vi "write_signal_hdf5.vi"(7 "Index":i32, 8 "error in":errorcluster, 10 "Save Path":path, 11 "Signal array":T2[](array[typedef])) -> (0 "error out":errorcluster, 3 "Signal Processing:":T4={"Integer Timestamp"=0, "Dust Event ID"=0, "Role ID"=enum."First_Detector", "Data"=[], "Signal Length"=0, "dt"=0.0, "Offset"=0.0, "Hardware ID"=enum."CSA 1"})   [LabVIEW 2013]
uses:
  <userlib>/Accelerator/User Interface/Controls/Post_Signal.ctl
  <userlib>/Accelerator/User Interface/Controls/Role ID.ctl
  <userlib>/Accelerator/User Interface/Controls/Hardware ID.ctl
  <userlib>/Accelerator/User Interface/Controls/Signal.ctl
  <vilib>/addons/h5labview/polymorph/H5D_write_var.vi
  <vilib>/addons/h5labview/H5Dataset.lvlib
  <vilib>/addons/h5labview/H5Attrib.lvlib
  <vilib>/addons/h5labview/H5File.lvlib
panel:
  out "concatenated string":string
  out "Role ID":T1
  # "Signal"
  # "Signal"
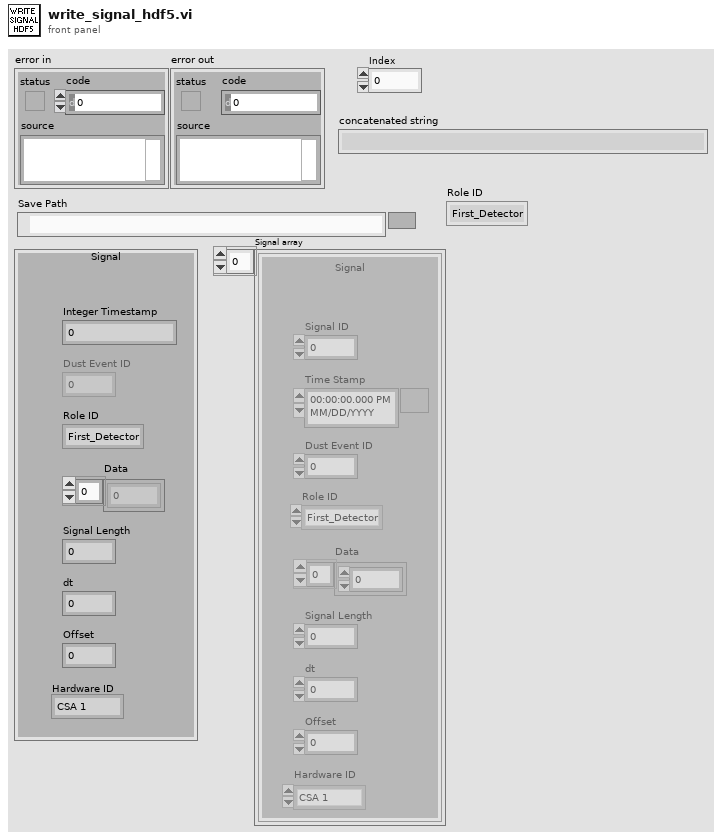
[diagram p1: front panel]
types:
  T1 = typedef "Role ID.ctl" = enum16{"First_Detector", "Second_Detector", "Third_Detector", "LeCroy_CH1", "LeCroy_CH2", "LeCroy_CH3", "LeCroy_CH4", "PSU", "DCS 1", "DCS 2"}
  T2 = typedef "Signal.ctl" = cluster{"Signal ID":i64, "Time Stamp":timestamp, "Dust Event ID":i64, "Role ID":T1, "Data":sgl[], "Signal Length":i32, "dt":sgl, "Offset":dbl, "Hardware ID":T3}
  T3 = typedef "Hardware ID.ctl" = enum16{"Unknown", "CSA 1", "CSA 2", "CSA 3", "CSA 4", "CSA 5", "CSA 6", "DCS 1", "DCS 2"}
  T4 = typedef "Post_Signal.ctl" = cluster{"Integer Timestamp":i64, "Dust Event ID":i64, "Role ID":T1, "Data":sgl[], "Signal Length":i32, "dt":sgl, "Offset":dbl, "Hardware ID":T3}
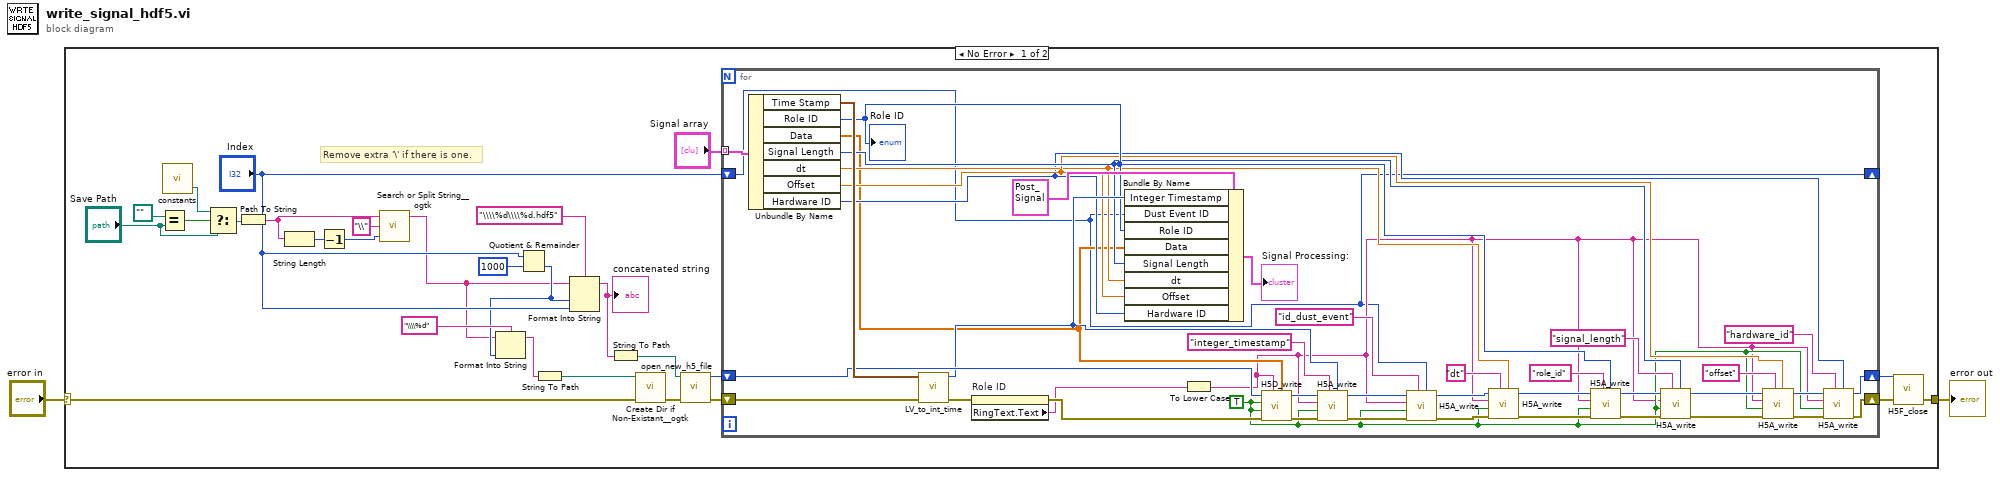
[diagram p0: block diagram]
diagram:
  n1 = case shown="No Error" "error in" {
    selector: "error in" -> [w3 w72]
    tunnel: [w5 w72] -> w1
    frame No Error {
      # "Remove extra '\\' if there is one."
      n2 = Equal?(x=path "" ("Save Path"), y="Save Path") -> (x = y?=w24:bool)
      n3 = call <userlib>:"constants.vi"() -> ("file path for Processed Signal .hdf5 files"=w4:path)  [unwired: 3 in, 2 out]
      n4 = Select(t=w4, s=w24, f="Save Path") -> (s? t:f=w26:path)
      n5 = Path To String(path=w26) -> (string=w9:string)
      n6 = String Length(string=w9) -> (length=w10:i32)
      n7 = Decrement(x=w10) -> (x-1=w11:i32)
      n8 = call <userlib>:"Search or Split String__ogtk.vi"("offset (0)"=w11, "search string/char (-)"="\\", "string"=w9) -> ("substring before match"=w8:string)  [unwired: 2 out]
      n9 = Quotient & Remainder(x="Index", y=1000) -> (floor(x/y)=w15:i32)  [unwired: 1 out]
      n10 = Format Into String(format string="\\\\%d", initial string=w8, w15) -> (resulting string=w16:string)  [unwired: 1 in, 1 out]
      n11 = String To Path(string=w16) -> (path=w13:path)
      n12 = Format Into String(format string="\\\\%d\\\\%d.hdf5", initial string=w8, w15, "Index") -> (resulting string=w19:string)  [unwired: 1 in, 1 out]
      "concatenated string" <- w19
      n13 = String To Path(string=w19) -> (path=w22:path)
      n14 = call <userlib>:"Create Dir if Non-Existant__ogtk.vi"("error in (no error)"=w3, "Directory Path"=w13) -> ("error out"=w14:errorcluster)  [unwired: 7 in, 2 out]
      n15 = call <userlib>:"open_new_h5_file.vi"("error in (no error)"=w14, "path"=w22) -> ("error out"=w28:errorcluster, "ref"=w27:i32)  [unwired: 8 in]
      n16 = for {
        tunnel: "Signal array" -> [w69] mode=indexing
        shift-right: [w43] -> w7
        shift-left: w28 -> [w68]
        shift-right: [w30] -> _
        shift-left: "Index" -> [w30]
        shift-right: [w42] -> w6
        shift-left: w27 -> [w65]
        w35 = TRUE ("preserve attribs?")
        n17 = Unbundle By Name(w69) -> ("Time Stamp"=w70:timestamp, "Role ID"=w54:T1, "Data"=w33:sgl[], "Signal Length"=w53:i32, "dt"=w36:sgl, "Offset"=w52:dbl, "Hardware ID"=w34:T3)
        "Role ID" <- w54
        n18 = call <userlib>:"LV_to_int_time.vi"("error in (no error)"=w68, "Time Stamp"=w70) -> ("error out"=w66:errorcluster, "Integer Time"=w60:i64)  [unwired: 7 in]
        n19 = property on="Role ID" class="Enum (strict)"(error in=w66) -> (error out=w64:errorcluster, "RingText.Text"=w32:string)  [unwired: 1 in, 1 out]
        n20 = Bundle By Name(cluster=T4 {"Integer Timestamp"=0, "Dust Event ID"=0, "Role ID"=enum."First_Detector", "Data"=[], "Signal Length"=0, "dt"=0.0, "Offset"=0.0, "Hardware ID"=enum."CSA 1"} ("Post_Signal 2"), "Integer Timestamp"=w60, "Dust Event ID"=w30, "Role ID"=w54, "Data"=w33, "Signal Length"=w53, "dt"=w36, "Offset"=w52, "Hardware ID"=w34) -> (→"Signal Processing:":T4)
        n21 = To Lower Case(string=w32) -> (all lower case string=w31:string)
        n22 = call-poly <vilib>:"H5D_write.vi"("data"=w33, "name"=w31, "error in (no error)"=w64, "overwrite?"=w35, "preserve attribs?"=w35, "ref"=w65) -> ("error out"=w62:errorcluster, "ref out"=w63:i32)  [unwired: 2 in]
        n23 = call <vilib>:"H5A_write.vi"("value"=w60, "attrib_name"="integer_timestamp", "error in (no error)"=w62, "overwrite? (F)"=w35, "obj_name"=w31, "ref"=w63) -> ("error out"=w48:errorcluster, "ref out"=w47:i32)  [unwired: 2 in]
        n24 = call <vilib>:"H5A_write.vi"("value"=w30, "attrib_name"="id_dust_event", "error in (no error)"=w48, "overwrite? (F)"=w35, "obj_name"=w31, "ref"=w47) -> ("error out"=w41:errorcluster, "ref out"=w38:i32)  [unwired: 2 in]
        n25 = call <vilib>:"H5A_write.vi"("value"=w36, "attrib_name"="dt", "error in (no error)"=w41, "overwrite? (F)"=w35, "obj_name"=w31, "ref"=w38) -> ("error out"=w40:errorcluster, "ref out"=w37:i32)  [unwired: 2 in]
        n26 = call <vilib>:"H5A_write.vi"("value"=w54, "attrib_name"="role_id", "error in (no error)"=w40, "overwrite? (F)"=w35, "obj_name"=w31, "ref"=w37) -> ("error out"=w49:errorcluster, "ref out"=w44:i32)  [unwired: 2 in]
        n27 = call <vilib>:"H5A_write.vi"("value"=w53, "attrib_name"="signal_length", "error in (no error)"=w49, "overwrite? (F)"=w35, "obj_name"=w31, "ref"=w44) -> ("error out"=w50:errorcluster, "ref out"=w45:i32)  [unwired: 2 in]
        n28 = call <vilib>:"H5A_write.vi"("value"=w52, "attrib_name"="offset", "error in (no error)"=w50, "overwrite? (F)"=w35, "obj_name"=w31, "ref"=w45) -> ("error out"=w51:errorcluster, "ref out"=w46:i32)  [unwired: 2 in]
        n29 = call <vilib>:"H5A_write.vi"("value"=w34, "attrib_name"="hardware_id", "error in (no error)"=w51, "overwrite? (F)"=w35, "obj_name"=w31, "ref"=w46) -> ("error out"=w43:errorcluster, "ref out"=w42:i32)  [unwired: 2 in]
      }
      n30 = call <vilib>:"H5F_close.vi"("error in (no error)"=w7, "ref"=w6) -> ("error out"=w5:errorcluster)  [unwired: 3 in]
    }
    frame Error {
    }
  }
  "error out" <- w1
